vi "Set LTS Stage Velocity Acceleration.vi"(8 "error in (no error)":errorcluster, 10 "Cluster in":T1, 11 "LTS Reference In":refnum<k24>) -> (0 "error out":errorcluster, 2 "Cluster out":T1, 3 "LTS Reference Out":refnum<k24>)   [LabVIEW 2014]
uses:
  Controls/Translation Stage Cluster.ctl
  General/Controls/Translation Stage Types.ctl
  C:/Project/SerialSectOCT/Software/Thorlabs.MotionControl.Controls.dll
  Thorlabs.MotionControl.Controls.dll
  C:/Project/SerialSectOCT/Software/Thorlabs.MotionControl.IntegratedStepperMotorsCLI.dll
  Thorlabs.MotionControl.IntegratedStepperMotorsCLI.dll
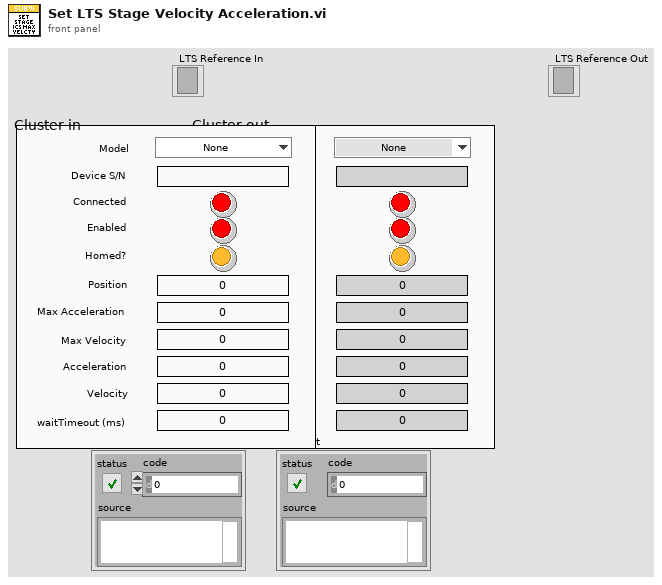
[diagram p1: front panel]
types:
  T1 = typedef "Translation Stage Cluster.ctl" = cluster{"Position":dbl, "Is.Enabled?":bool, "Is.Connected?":bool, "Device SN":string, "AccelerationMaximum":dbl, "VelocityMaximum":dbl, "Acceleration":dbl, "Velocity":dbl, "waitTimeout (ms)":i32, "Model":T2, "Is.Homed?":bool}
  T2 = typedef "Translation Stage Types.ctl" = enum16{"None", "Thorlabs LTS", "Thorlabs MLJ"}
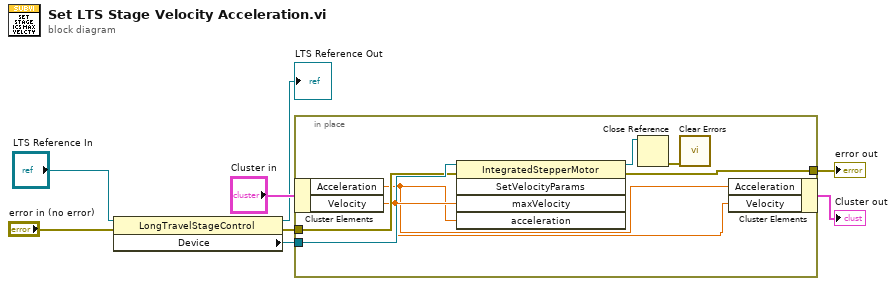
[diagram p0: block diagram]
diagram:
  n1 = property class="LongTravelStageControl"(reference="LTS Reference In", error in="error in (no error)") -> (reference out=→"LTS Reference Out":refnum<k24>, error out=w2:errorcluster, "Device"=w1:refnum<k24>)
  n2 = in-place {
    in-place-border: w1 -> [w15]
    in-place-border: w2 -> [w14]
    in-place-border: [w13] -> w6
    n3 = in-place-cluster #1("Cluster in") -> ("Acceleration"=w9:dbl, "Velocity"=w10:dbl)
    n4 = invoke class="IntegratedStepperMotor" method="SetVelocityParams"(reference=w15, error in=w14, "maxVelocity"=w10, "acceleration"=w9) -> (reference out=w11:refnum<k24>, error out=w13:errorcluster)  [unwired: 1 in, 3 out]
    n5 = Close Reference(reference=w11) -> (error out=w12:errorcluster)  [unwired: 1 in]
    n6 = call <vilib>:"Clear Errors.vi"("error in (no error)"=w12) -> ()  [unwired: 5 in, 2 out]
    n7 = in-place-cluster #1("Acceleration"=w9, "Velocity"=w10) -> (→"Cluster out":T1)
  }
  "error out" <- w6
